vi "RTS Main Door Opener.vi"(4 "Station #":u8=1 min=1 max=8 step=1, 5 "Relay Number":u8=1 min=1 max=3 step=1, 6 "Current Status":string[](array[string]), 7 "Array Size":i32, 8 "Error In":errorcluster, 11 "Station 1-8 Data":T1={"Station Freezer"={"Time Count (s)"=0.0, "Status"="", "Door State"=FALSE, "Delay"=TRUE, "Chamber 1-1"=[], "Index"=0, "Delay Status"=""}, "Station Cab"={"Time Count (s)"=0.0, "Status"="", "Door State"=FALSE, "Delay"=TRUE, "Chamber 1-1"=[], "Index"=0, "Delay Status"=""}, "Station Slide"={"Time Count (s)"=0.0, "Status"="", "Door State"=FALSE, "Delay"=TRUE, "Chamber 1-1"=[], "Index"=0, "Delay Status"=""}, "1st Complete"=FALSE, "2nd Complete"=FALSE, "3rd Complete"=FALSE} {"Station Slide"."Chamber 1-1"."Start Time" format="%<%X\n%x>T"; "Station Slide"."Chamber 1-1"."End Time" format="%<%X\n%x>T"; "Station Slide"."Time Count (s)" format="%.2f"; "Station Cab"."Chamber 1-1"."Start Time" format="%<%X\n%x>T"; "Station Cab"."Chamber 1-1"."End Time" format="%<%X\n%x>T"; "Station Cab"."Time Count (s)" format="%.2f"; "Station Freezer"."Chamber 1-1"."Start Time" format="%<%X\n%x>T"; "Station Freezer"."Chamber 1-1"."End Time" format="%<%X\n%x>T"; "Station Freezer"."Time Count (s)" format="%.2f"}) -> (0 "Error Out":errorcluster, 3 "Station Cluster":T1={"Station Freezer"={"Time Count (s)"=0.0, "Status"="", "Door State"=FALSE, "Delay"=TRUE, "Chamber 1-1"=[], "Index"=0, "Delay Status"=""}, "Station Cab"={"Time Count (s)"=0.0, "Status"="", "Door State"=FALSE, "Delay"=TRUE, "Chamber 1-1"=[], "Index"=0, "Delay Status"=""}, "Station Slide"={"Time Count (s)"=0.0, "Status"="", "Door State"=FALSE, "Delay"=TRUE, "Chamber 1-1"=[], "Index"=0, "Delay Status"=""}, "1st Complete"=FALSE, "2nd Complete"=FALSE, "3rd Complete"=FALSE} {"Station Slide"."Chamber 1-1"."Start Time" format="%<%X\n%x>T"; "Station Slide"."Chamber 1-1"."End Time" format="%<%X\n%x>T"; "Station Slide"."Time Count (s)" format="%.2f"; "Station Cab"."Chamber 1-1"."Start Time" format="%<%X\n%x>T"; "Station Cab"."Chamber 1-1"."End Time" format="%<%X\n%x>T"; "Station Cab"."Time Count (s)" format="%.2f"; "Station Freezer"."Chamber 1-1"."Start Time" format="%<%X\n%x>T"; "Station Freezer"."Chamber 1-1"."End Time" format="%<%X\n%x>T"; "Station Freezer"."Time Count (s)" format="%.2f"})   [LabVIEW 2016]
uses:
  Type Definitions/RTS Station Relay Ops.ctl
  Type Definitions/RTS Door Opener Indicator.ctl
  Type Definitions/RTS Door Ops Client.ctl
  Type Definitions/RTS Door Opening Schedule.ctl
  Type Definitions/RTS Door Ops Sequence.ctl
panel:
  # "Chamber Conditions:"
  # "Chamber Conditions:"
  # "Chamber Conditions:"
  # "Chamber Conditions:"
  # "Chamber Conditions:"
  # "Chamber Conditions:"
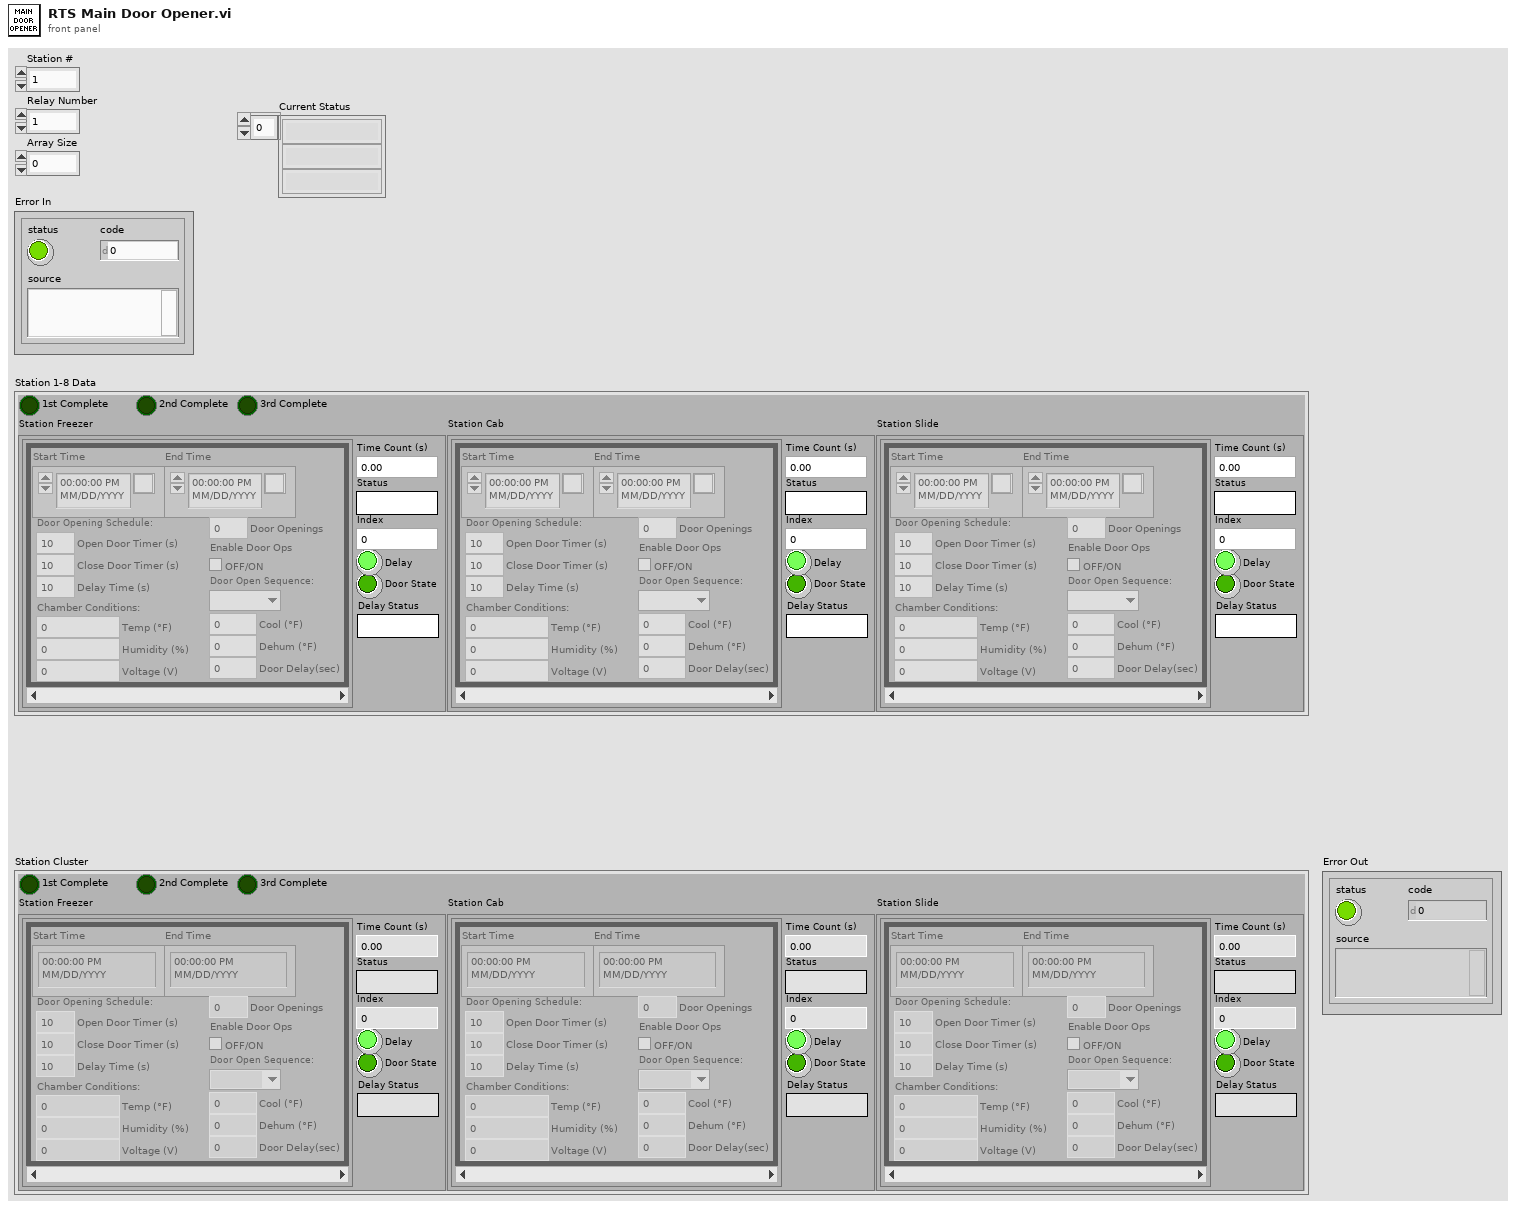
[diagram p1: front panel]
types:
  T1 = typedef "RTS Station Relay Ops.ctl" = cluster{"Station Freezer":T2, "Station Cab":T2, "Station Slide":T2, "1st Complete":bool, "2nd Complete":bool, "3rd Complete":bool}
  T2 = typedef "RTS Door Opener Indicator.ctl" = cluster{"Time Count (s)":dbl, "Status":string, "Door State":bool, "Delay":bool, "Chamber 1-1":T3[], "Index":i32, "Delay Status":string}
  T3 = typedef "RTS Door Ops Client.ctl" = cluster{"End Time":timestamp, "Start Time":timestamp, "Door Opening Schedule:":T4, "Enable Door Ops":bool, "Door Openings":u32, "Temp (°F)":dbl, "Humidity (%)":dbl, "Voltage (V)":dbl, "Door Open Sequence:":T5, "Door Delay(sec)":dbl, "Dehum (°F)":dbl, "Cool (°F)":dbl}
  T4 = typedef "RTS Door Opening Schedule.ctl" = cluster{"Open Door Timer (s)":dbl, "Delay Time (s)":dbl, "Close Door Timer (s)":dbl}
  T5 = typedef "RTS Door Ops Sequence.ctl" = enum16{"", "1st", "2nd", "3rd"}
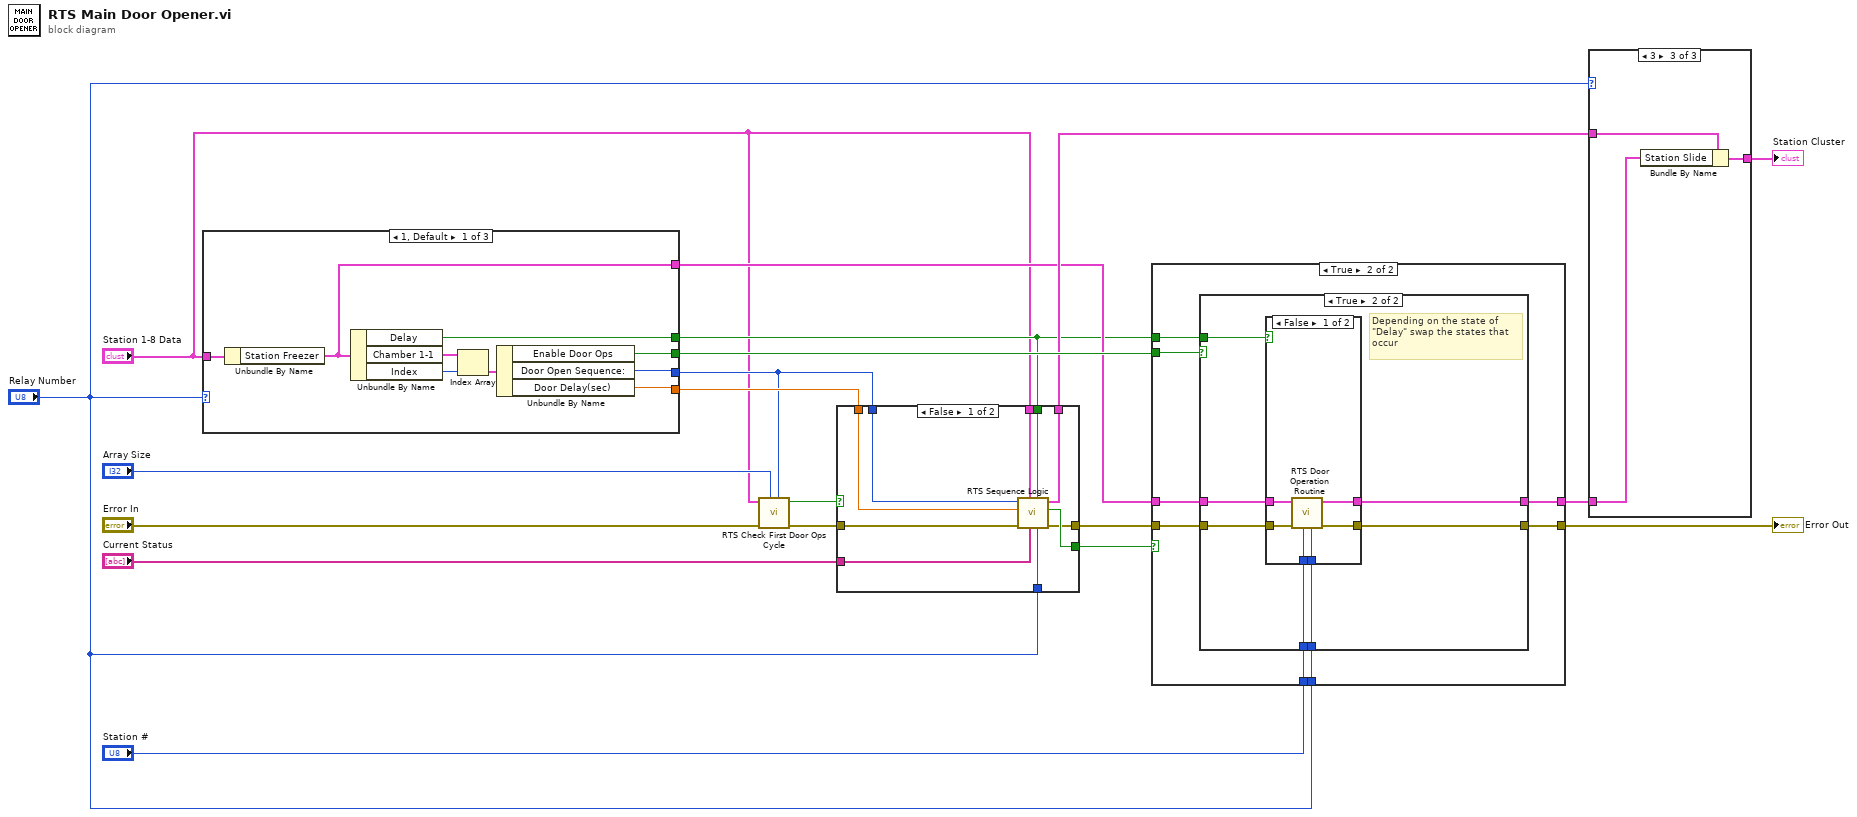
[diagram p0: block diagram]
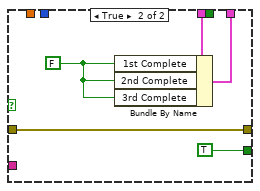
[diagram p2: hidden frame]
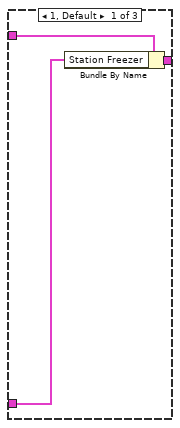
[diagram p3: hidden frame]
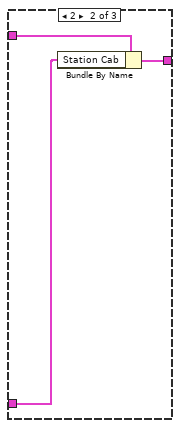
[diagram p4: hidden frame]
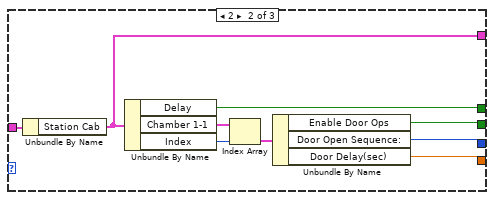
[diagram p5: hidden frame]
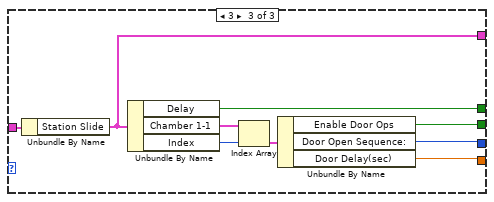
[diagram p6: hidden frame]
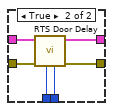
[diagram p9: hidden frame]
diagram:
  n1 = case shown="1, Default" "Relay Number" {
    tunnel: [w28 w34 w43] -> w10
    tunnel: [w24 w33 w42] -> w17
    tunnel: [w23 w31 w40] -> w4
    tunnel: [w22 w32 w41] -> w15
    tunnel: "Station 1-8 Data" -> [w21 w30 w39]
    tunnel: [w20 w29 w38] -> w12
    frame 1, Default {
      n2 = Unbundle By Name(w21) -> ("Station Freezer"=w20:T2)
      n3 = Unbundle By Name(w20) -> ("Delay"=w28:bool, "Chamber 1-1"=w27:T3[], "Index"=w26:i32)
      n4 = Index Array(array=w27, index=w26) -> (element=w25:T3)
      n5 = Unbundle By Name(w25) -> ("Enable Door Ops"=w24:bool, "Door Open Sequence:"=w23:T5, "Door Delay(sec)"=w22:dbl)
    }
    frame 2 {
      n6 = Unbundle By Name(w30) -> ("Station Cab"=w29:T2)
      n7 = Unbundle By Name(w29) -> ("Delay"=w34:bool, "Chamber 1-1"=w37:T3[], "Index"=w36:i32)
      n8 = Index Array(array=w37, index=w36) -> (element=w35:T3)
      n9 = Unbundle By Name(w35) -> ("Enable Door Ops"=w33:bool, "Door Open Sequence:"=w31:T5, "Door Delay(sec)"=w32:dbl)
    }
    frame 3 {
      n10 = Unbundle By Name(w39) -> ("Station Slide"=w38:T2)
      n11 = Unbundle By Name(w38) -> ("Delay"=w43:bool, "Chamber 1-1"=w46:T3[], "Index"=w45:i32)
      n12 = Index Array(array=w46, index=w45) -> (element=w44:T3)
      n13 = Unbundle By Name(w44) -> ("Enable Door Ops"=w42:bool, "Door Open Sequence:"=w40:T5, "Door Delay(sec)"=w41:dbl)
    }
  }
  n14 = call "RTS Check First Door Ops Cycle.vi"("Door Open Sequence:"=w4, "Array Size"="Array Size", "error in (no error)"="Error In", "Station 1-8 Data in"="Station 1-8 Data") -> ("error out"=w6:errorcluster, "First Cycle Complete"=w1:bool)  [unwired: 6 in]
  n15 = case shown="False" w1 {
    tunnel: [w56 TRUE ("Run Door Op Sequence")] -> w16
    tunnel: w15 -> [w55 _]
    tunnel: [w54 w61] -> w14
    tunnel: [w53 w58] -> w13
    tunnel: w10 -> [w52 _]
    tunnel: "Relay Number" -> [w51 _]
    tunnel: w6 -> [w50 w61]
    tunnel: w4 -> [w49 _]
    tunnel: "Current Status" -> [w48 _]
    tunnel: "Station 1-8 Data" -> [w47 w59]
    frame False {
      n16 = call "RTS Sequence Logic.vi"("Relay Number"=w51, "Delay"=w52, "Current Status"=w48, "Station 1-8 Data in"=w47, "error in (no error)"=w50, "Door Open Delay(sec)"=w55, "Door Open Sequence:"=w49) -> ("error out"=w54:errorcluster, "Run Door Op Sequence"=w56:bool, "Station 1-8 Data out"=w53:T1)  [unwired: 2 in]
    }
    frame True {
      w57 = FALSE ("1st Complete")
      n17 = Bundle By Name(cluster=w59, "1st Complete"=w57, "2nd Complete"=w57, "3rd Complete"=w57) -> (w58:T1)
    }
  }
  n18 = case shown="True" w16 {
    tunnel: w10 -> [_ w71]
    tunnel: [w63 w70] -> w19
    tunnel: [w62 w69] -> w18
    tunnel: w12 -> [w63 w68]
    tunnel: w17 -> [_ w67]
    tunnel: w14 -> [w62 w66]
    tunnel: "Station #" -> [_ w64]
    tunnel: "Relay Number" -> [_ w65]
    frame False {
    }
    frame True {
      n19 = case shown="True" w67 {
        tunnel: w71 -> [_ w80]
        tunnel: w68 -> [w73 w79]
        tunnel: w66 -> [w72 w78]
        tunnel: [w73 w77] -> w70
        tunnel: [w72 w76] -> w69
        tunnel: w65 -> [_ w74]
        tunnel: w64 -> [_ w75]
        frame False {
        }
        frame True {
          # "Depending on the state of\n\"Delay\" swap the states that \noccur"
          n20 = case shown="False" w80 {
            tunnel: w79 -> [w86 w92]
            tunnel: [w85 w91] -> w77
            tunnel: [w84 w89] -> w76
            tunnel: w78 -> [w83 w90]
            tunnel: w75 -> [w82 w88]
            tunnel: w74 -> [w81 w87]
            frame False {
              n21 = call "RTS Door Operation Routine.vi"("Relay Number"=w81, "Station #"=w82, "Error In"=w83, "Door Opening Controller Input"=w86) -> ("Error Out"=w84:errorcluster, "Door Opening Controller Output"=w85:T2)  [unwired: 6 in]
            }
            frame True {
              n22 = call "RTS Door Delay.vi"("Relay Number"=w87, "Station #"=w88, "Error In"=w90, "Door Opening Controller Input"=w92) -> ("Error Out"=w89:errorcluster, "Door Opening Controller Output"=w91:T2)  [unwired: 6 in]
            }
          }
        }
      }
    }
  }
  "Error Out" <- w18
  n23 = case shown="3" "Relay Number" {
    tunnel: w19 -> [w94 w96 w99]
    tunnel: w13 -> [w95 w98 w101]
    tunnel: [w93 w97 w100] -> w11
    frame 1, Default {
      n24 = Bundle By Name(cluster=w95, "Station Freezer"=w94) -> (w93:T1)
    }
    frame 2 {
      n25 = Bundle By Name(cluster=w98, "Station Cab"=w96) -> (w97:T1)
    }
    frame 3 {
      n26 = Bundle By Name(cluster=w101, "Station Slide"=w99) -> (w100:T1)
    }
  }
  "Station Cluster" <- w11
